vi "Thermometer (Demo).vi"(1 "单位（0：摄氏度）":u16(ring) items=["摄氏", "华氏"]) -> (0 "温度值":dbl(slide) scale=0.0..100.0)   [LabVIEW 2012]
doc: "该VI可模拟通过DAQ BNC-2120接线盒上的温度传感器测量温度。\n\n如已有DAQ板卡连接至BNC-2120且在MAX中已配置了系统，请使用“温度计”VI替代该VI。"
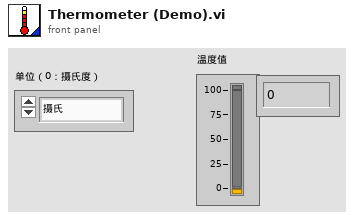
[diagram p1: front panel]
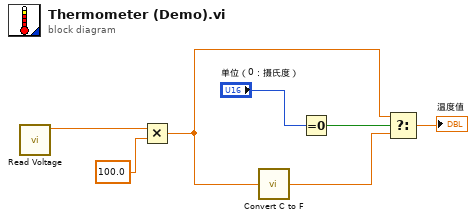
[diagram p0: block diagram]
diagram:
  n1 = call "Read Voltage.vi"() -> ("电压"=w4:dbl)  [unwired: 8 in, 1 out]
  n2 = Multiply ("乘")(x=w4, y=100.0) -> (x*y=w5:dbl)
  n3 = call "Convert C to F.vi"("摄氏温标"=w5) -> ("华氏温标"=w7:dbl)
  n4 = Equal To 0? ("等于0？")(x="单位（0：摄氏度）") -> (x = 0?=w1:bool)
  n5 = Select ("选择")(t=w5, s=w1, f=w7) -> (s? t:f=→"温度值":dbl)
